vi "NATS Server Stop Windows.vi"(8 "error in":errorcluster) -> (0 "error out":errorcluster)   [LabVIEW 2024, in "NATS Infrastructure.lvlib"]
doc: "Starts NATS server on Windows machines."
uses:
  NATS Infrastructure.lvlib
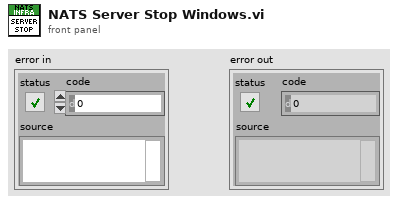
[diagram p1: front panel]
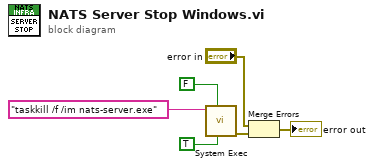
[diagram p0: block diagram]
diagram:
  n1 = call <vilib>:"System Exec.vi"("run minimized? (F)"=TRUE, "wait until completion? (T)"=FALSE, "command line"="taskkill /f /im nats-server.exe") -> ("error out"=w2:errorcluster)  [unwired: 5 in, 3 out]
  n2 = Merge Errors("error in", w2) -> (→"error out":errorcluster)
